vi "_RT_CtrlLoop_Laser_Read_VISA.vi"(8 "error in (no error)":errorcluster, 10 "Comm Str":string, 11 "VISA resource In":refnum<visa-resource-name>) -> (0 "error out":errorcluster, 2 "Response Str":string, 3 "VISA resource Out":refnum<visa-resource-name>)   [LabVIEW 2018]
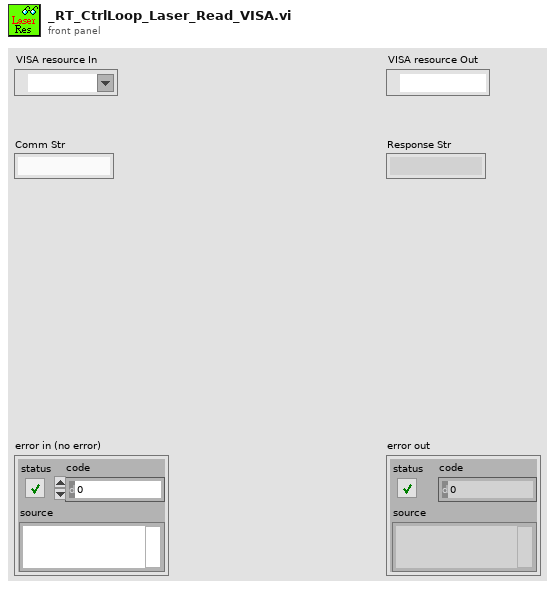
[diagram p1: front panel]
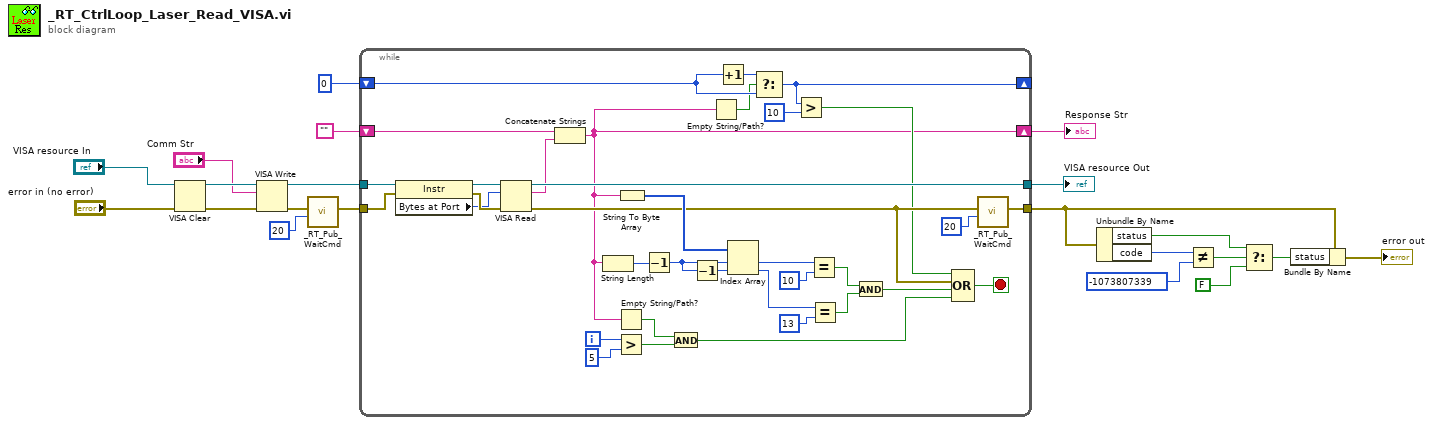
[diagram p0: block diagram]
diagram:
  n1 = VISA Clear(VISA resource name="VISA resource In", error in (no error)="error in (no error)") -> (VISA resource name out=w17:refnum<visa-resource-name>, error out=w14:errorcluster)
  n2 = VISA Write(VISA resource name=w17, write buffer="Comm Str", error in (no error)=w14) -> (VISA resource name out=w16:refnum<visa-resource-name>, error out=w5:errorcluster)  [unwired: 1 out]
  n3 = call "_RT_Pub_WaitCmd.vi"("milliseconds to wait"=u32 20, "error in (no error)"=w5) -> ("error out"=w4:errorcluster)  [unwired: 9 in]
  n4 = while {
    shift-right: [w23] -> w20
    shift-left: "" -> [w56]
    tunnel: [w55] -> w19
    tunnel: [w30] -> w10
    tunnel: w16 -> [w42]
    tunnel: w4 -> [w41]
    shift-right: [w26] -> _
    shift-left: 0 -> [w27]
    i -> [w37]
    stop <- w22 stop-if-true
    n5 = property class="Instr"(reference=w42, error in=w41) -> (reference out=w40:refnum<visa-resource-name>, error out=w39:errorcluster, "Bytes at Port"=w38:u32)
    n6 = VISA Read(VISA resource name=w40, byte count=w38, error in (no error)=w39) -> (VISA resource name out=w55:refnum<visa-resource-name>, read buffer=w53:string, error out=w31:errorcluster)  [unwired: 1 out]
    n7 = Concatenate Strings(w56, w53) -> (w23:string)
    n8 = String Length(string=w23) -> (length=w43:i32)
    n9 = Empty String/Path?(string/path=w23) -> (empty?=w35:bool)
    n10 = Greater?(x=w37, y=5) -> (0:w34:bool)
    n11 = String To Byte Array(string=w23) -> (unsigned byte array=w54:u8[])
    n12 = Decrement(x=w43) -> (x-1=w50:i32)
    n13 = And(x=w35, y=w34) -> (x .and. y?=w33:bool)
    n14 = Decrement(x=w50) -> (x-1=w49:i32)
    n15 = Empty String/Path?(string/path=w23) -> (empty?=w24:bool)
    n16 = Increment(x=w27) -> (x+1=w29:i32)
    n17 = Index Array(array=w54, index #1=w50, index #2=w49) -> (element #1=w52:u8, element #2=w48:u8)
    n18 = Select(t=w29, s=w24, f=w27) -> (s? t:f=w26:i32)
    n19 = Greater?(x=w26, y=10) -> (0:w25:bool)
    n20 = Equal?(x=w52, y=u8 10) -> (x = y?=w46:bool)
    n21 = Equal?(x=w48, y=u8 13) -> (x = y?=w45:bool)
    n22 = And(x=w46, y=w45) -> (x .and. y?=w44:bool)
    n23 = Compound Arithmetic op=OR(w25, w31, w44, w33) -> (w22:bool)
    n24 = call "_RT_Pub_WaitCmd.vi"("milliseconds to wait"=u32 20, "error in (no error)"=w31) -> ("error out"=w30:errorcluster)  [unwired: 9 in]
  }
  "VISA resource Out" <- w19
  "Response Str" <- w20
  n25 = Unbundle By Name(w10) -> ("status"=w8:bool, "code"=w13:i32)
  n26 = Not Equal?(x=w13, y=-1073807339) -> (x != y?=w9:bool)
  n27 = Select(t=w8, s=w9, f=FALSE) -> (s? t:f=w6:bool)
  n28 = Bundle By Name(cluster=w10, "status"=w6) -> (→"error out":errorcluster)
